vi "Create Generic 3 Queues.vi"(8 "error in (no error)":errorcluster, 11 "name":string="selectspectrum") -> (0 "error out":errorcluster, 3 "Message Queues":T1)   [LabVIEW 2022 SP3, in "Front Panel Message Queue.lvlib"]
doc: "This VI creates and initializes all the message queues for your application. If your application requires more than one message queue, right-click the \"Message Queues\" constant above and select Open Type Def. Add the new Message Queue(s) to the type definition, then initialize them in this VI."
uses:
  Front Panel Message Queue.lvlib
  Enqueue Message (Single).vi
  Message Cluster.ctl
  load 3 Messages Queues.ctl
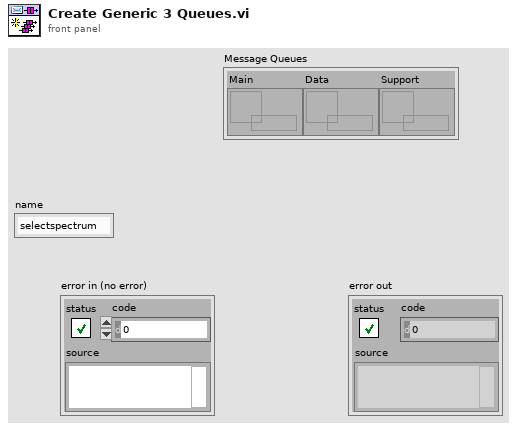
[diagram p1: front panel]
types:
  T1 = typedef "Front Panel Message Queue.lvlib/load 3 Messages Queues.ctl" = cluster{"Main":refnum<queue>, "Data":refnum<queue>, "Support":refnum<queue>}
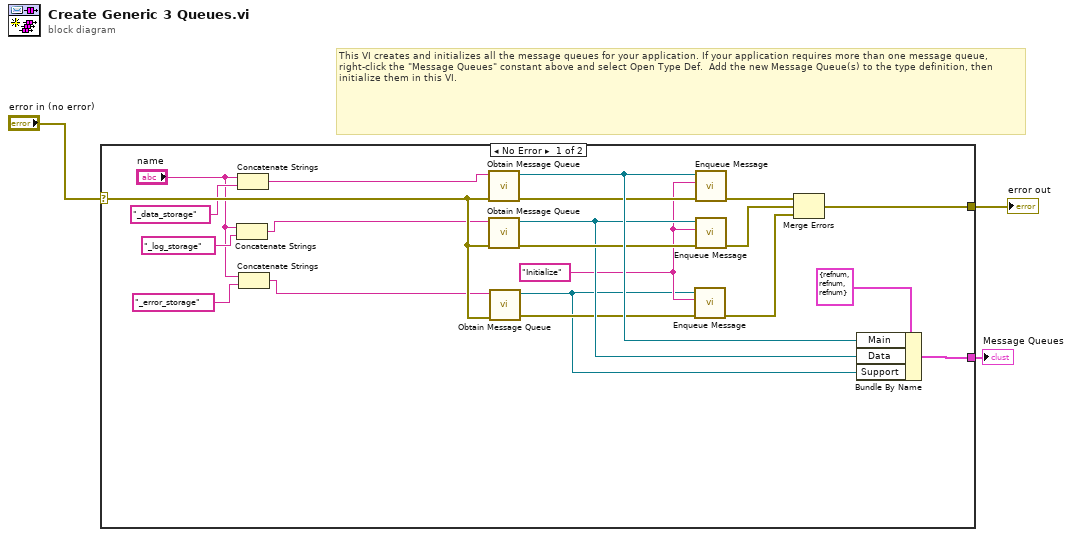
[diagram p0: block diagram]
diagram:
  # "This VI creates and initializes all the message queues for your application. If your application requires more than one message queue, right-click the \"Message Queues\" constant above and select Open Type Def.  Add the new Message Queue(s) to the type definition, then initialize them in this VI."
  n1 = case shown="No Error" "error in (no error)" {
    selector: "error in (no error)" -> [w15 w25]
    tunnel: [w19 w25] -> w3
    tunnel: [w24 _] -> w1
    frame No Error {
      w13 = "Initialize" ("Message")
      n2 = Concatenate Strings("name", "_log_storage" ("string")) -> (w7:string)
      n3 = Concatenate Strings("name", "_data_storage" ("string")) -> (w4:string)
      n4 = Concatenate Strings("name", "_error_storage" ("string")) -> (w9:string)
      n5 = call "Obtain Message Queue.vi"("error in (no error)"=w15, "name"=w4) -> ("error out"=w22:errorcluster, "Message Queue"=w23:refnum<queue>)  [unwired: 8 in]
      n6 = call "Obtain Message Queue.vi"("error in (no error)"=w15, "name"=w7) -> ("error out"=w21:errorcluster, "Message Queue"=w17:refnum<queue>)  [unwired: 8 in]
      n7 = call "Obtain Message Queue.vi"("error in (no error)"=w15, "name"=w9) -> ("error out"=w14:errorcluster, "Message Queue"=w12:refnum<queue>)  [unwired: 8 in]
      n8 = call-poly "Enqueue Message.vi"("error in (no error)"=w14, "Message"=w13, "Message Queue"=w12) -> ("error out"=w11:errorcluster)  [unwired: 7 in, 1 out]
      n9 = call-poly "Enqueue Message.vi"("error in (no error)"=w22, "Message"=w13, "Message Queue"=w23) -> ("error out"=w20:errorcluster)  [unwired: 7 in, 1 out]
      n10 = call-poly "Enqueue Message.vi"("error in (no error)"=w21, "Message"=w13, "Message Queue"=w17) -> ("error out"=w18:errorcluster)  [unwired: 7 in, 1 out]
      n11 = Merge Errors(w20, w18, w11) -> (w19:errorcluster)
      n12 = Bundle By Name(cluster=T1 {"Main"=refnum, "Data"=refnum, "Support"=refnum} ("Message Queues"), "Main"=w23, "Data"=w17, "Support"=w12) -> (w24:T1)
    }
    frame Error {
    }
  }
  "error out" <- w3
  "Message Queues" <- w1
